vi "HW_GEN - Write Channel Default Parameters to XML File.vi"(8 "error in":errorcluster caption="错误输入（无错误）", 9 "Dflt Units[]":string, 10 "ChanType":string="AI_QX", 11 "path to XML document":path=path "E:/00. 系统集成/!00000/11所 热气台等/SourceCodes/Builds/Files/CHdef.xml" caption="XML文档路径") -> (0 "错误输出":errorcluster)   [LabVIEW 2016]
uses:
  <vilib>/xml/Load XML File.vi
  <vilib>/xml/Close Reference(Node).vi
  <vilib>/xml/NI_XML.lvlib
  <resource>/objmgr/DOMUserDefRef.rc
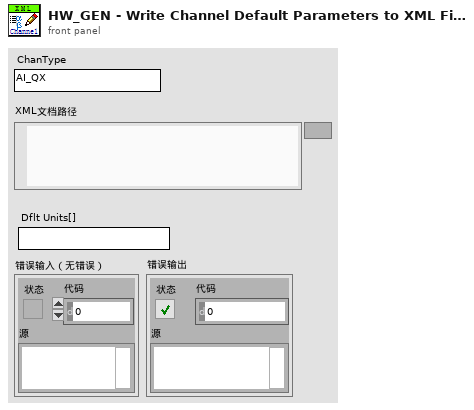
[diagram p1: front panel]
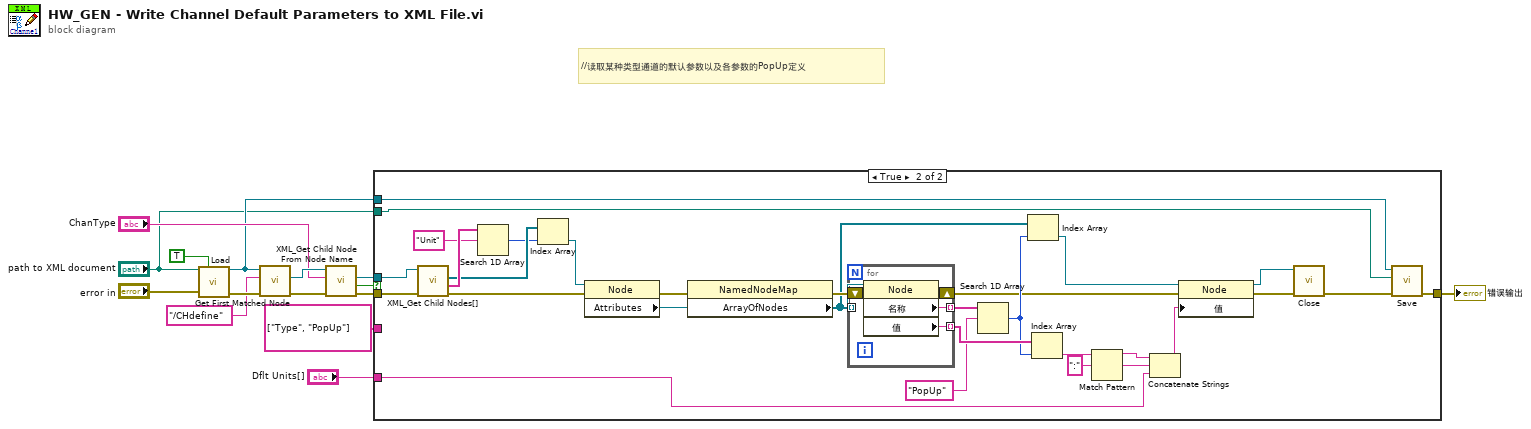
[diagram p0: block diagram]
diagram:
  # "//读取某种类型通道的默认参数以及各参数的PopUp定义"
  n1 = call-poly <vilib>:"Load.vi"("path to XML document"="path to XML document", "preserve whitespace (True)"=TRUE, "error in (no error)"="error in") -> ("DOM document out"=w2:refnum<k20>, "error out"=w14:errorcluster)  [unwired: 10 in, 1 out]
  n2 = call <vilib>:"Get First Matched Node.vi"("error in (no error)"=w14, "XPath expression"="/CHdefine", "node in"=w2) -> ("error out"=w11:errorcluster, "node result"=w12:refnum<k20>)  [unwired: 6 in, 1 out]
  n3 = call "XML_Get Child Node From Node Name.vi"("error in"=w11, "NodeName"="ChanType", "ref in"=w12) -> ("错误输出"=w6:errorcluster, "find?"=w8:bool, "subNode out"=w7:refnum<k20>)  [unwired: 6 in]
  n4 = case shown="True" w8 {
    tunnel: w7 -> [_ w44]
    tunnel: w6 -> [w16 w45]
    tunnel: string[] ["Type", "PopUp"] ("AttributeNames") -> [_ _]
    tunnel: [w16 w23] -> w4
    tunnel: "Dflt Units[]" -> [_ w24]
    tunnel: w2 -> [_ w21]
    tunnel: "path to XML document" -> [_ w20]
    frame False {
    }
    frame True {
      w25 = ":" ("regular expression")
      n5 = call "XML_Get Child Nodes[].vi"("错误输入（无错误）"=w45, "ref in"=w44) -> ("错误输出"=w33:errorcluster, "NodeNames[]"=w43:string[], "ElementChildNod[]"=w41:refnum<k20>[])  [unwired: 6 in, 1 out]
      n6 = Search 1D Array(1D array=w43, element="Unit") -> (index of element=w40:i32)  [unwired: 1 in]
      n7 = Index Array(array=w41, index=w40) -> (element=w34:refnum<k20>)
      n8 = property on="属性节点" class="Node"(reference=w34, error in=w33) -> (error out=w38:errorcluster, "Attributes"=w39:refnum<k20>)  [unwired: 1 out]
      n9 = property on="属性节点" class="NamedNodeMap"(reference=w39, error in=w38) -> (error out=w37:errorcluster, "ArrayOfNodes"=w31:refnum<k20>[])  [unwired: 1 out]
      n10 = for {
        tunnel: w31 -> [w50] mode=indexing
        tunnel: [w49] -> w36 mode=indexing
        tunnel: [w48] -> w35 mode=indexing
        shift-right: [w46] -> w28
        shift-left: w37 -> [w47]
        n11 = property on="属性节点" class="Node"(reference=w50, error in=w47) -> (error out=w46:errorcluster, "名称"=w49:string, "值"=w48:string)  [unwired: 1 out]
      }
      n12 = Search 1D Array(1D array=w36, element="PopUp" ("名称")) -> (index of element=w30:i32)  [unwired: 1 in]
      n13 = Index Array(array=w31, index=w30) -> (element=w29:refnum<k20>)
      n14 = Index Array(array=w35, index=w30) -> (element=w27:string)
      n15 = Match Pattern(string=w27, regular expression=w25) -> (before substring=w26:string)  [unwired: 1 in, 3 out]
      n16 = Concatenate Strings(w26, w25, w24) -> (w22:string)
      n17 = property on="属性节点" class="Node"(reference=w29, error in=w28, "值"=w22) -> (reference out=w19:refnum<k20>, error out=w18:errorcluster)
      n18 = call-poly <vilib>:"Close.vi"("error in (no error)"=w18, "node"=w19) -> ("error out"=w17:errorcluster)  [unwired: 7 out]
      n19 = call <vilib>:"Save.vi"("error in (no error)"=w17, "XML file path"=w20, "DOM document in"=w21) -> ("error out"=w23:errorcluster)  [unwired: 6 in, 2 out]
    }
  }
  "错误输出" <- w4
